vi "Set_Window_Saved.vi"(1 "Saved":bool, 2 "VI Path":path) -> ()   [LabVIEW 2011]
doc: "This VI appends a \"*\" character to the window title if the \"Saved\" parameter is true, and removes the \"*\" character if the \"Saved\" parameter is false. The window is given by the \"VI Path\" parameter."
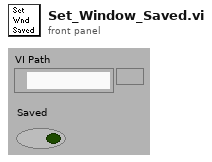
[diagram p1: front panel]
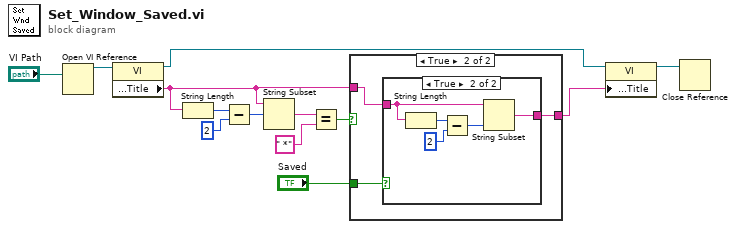
[diagram p0: block diagram]
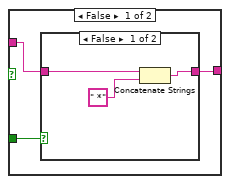
[diagram p2: hidden frame]
diagram:
  n1 = Open VI Reference(vi path="VI Path") -> (vi reference=w11:refnum<vi>)  [unwired: 2 in, 4 out]
  n2 = property class="VI"(reference=w11) -> (reference out=w10:refnum<vi>, "Front Panel.Title"=w3:string)  [unwired: 1 in, 1 out]
  n3 = String Length(string=w3) -> (length=w9:i32)
  n4 = Subtract(x=w9, y=2) -> (x-y=w7:i32)
  n5 = String Subset(string=w3, offset (0)=w7) -> (substring=w6:string)  [unwired: 1 out]
  n6 = Equal?(x=w6, y=" *") -> (x = y?=w4:bool)
  n7 = case shown="True" w4 {
    tunnel: w3 -> [w14 w22]
    tunnel: "Saved" -> [w16 w23]
    tunnel: [w15 w21] -> w1
    frame False {
      n8 = case shown="False" w16 {
        tunnel: [w18 w20] -> w15
        tunnel: w14 -> [w19 w20]
        frame False {
          n9 = Concatenate Strings(w19, " *" ("string")) -> (w18:string)
        }
        frame True {
        }
      }
    }
    frame True {
      n10 = case shown="True" w23 {
        tunnel: w22 -> [w24 w26]
        tunnel: [w24 w25] -> w21
        frame False {
        }
        frame True {
          n11 = String Length(string=w26) -> (length=w29:i32)
          n12 = Subtract(x=w29, y=2) -> (x-y=w28:i32)
          n13 = String Subset(string=w26, length (rest)=w28) -> (substring=w25:string)  [unwired: 1 out]
        }
      }
    }
  }
  n14 = property class="VI"(reference=w10, "Front Panel.Title"=w1) -> (reference out=w13:refnum<vi>)  [unwired: 1 in, 1 out]
  n15 = Close Reference(reference=w13) -> ()  [unwired: 1 in, 1 out]
